vi "Get IData Sink.vi"(11 "Data Logger Actor in":refnum<class "Data Logger Actor.lvclass">) -> (2 "IData Sink":refnum<class "IData Sink.lvclass">, 3 "Data Logger Actor out":refnum<class "Data Logger Actor.lvclass">)   [LabVIEW 2024, in "Data Logger Actor.lvlib" / "Data Logger Actor.lvclass"]
uses:
  Data Logger Actor.lvclass
  Data Sink/IData Sink/IData Sink.lvclass
  Data Logger Actor.lvclass/Data Logger Actor.ctl
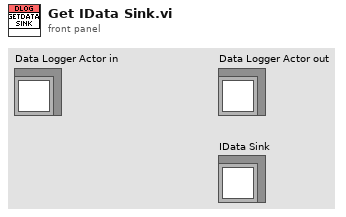
[diagram p1: front panel]
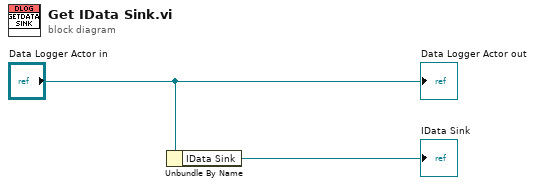
[diagram p0: block diagram]
diagram:
  n1 = Unbundle By Name("Data Logger Actor in") -> ("IData Sink"=→"IData Sink":refnum<class "IData Sink.lvclass">)
  "Data Logger Actor out" <- "Data Logger Actor in"
